vi "Create File Path.vi"(5 "system directory type":T2 caption="시스템 디렉토리 타입" items=["사용자 홈"=0, "사용자 데스크탑"=1, "사용자 문서"=2, "사용자 어플리케이션 데이터"=3, "사용자 환경"=4, "사용자 임시"=5, "퍼블릭 문서"=6, "퍼블릭 어플리케이션 데이터"=7, "퍼블릭 환경"=8, "퍼블릭 캐시"=13, "시스템 코어 라이브러리"=9, "시스템 설치된 라이브러리"=10, "어플리케이션 파일"=11, "부팅 볼륨 루트"=12], 6 "파일타입":T1, 7 "항목":T3=enum."경로생성", 8 "에러 입력":errorcluster caption="에러 입력(에러 없음)", 10 "문자열 in":string, 11 "폴더명 in":path) -> (0 "error out":errorcluster, 1 "파일존재?":bool, 2 "문자열 out":string, 3 "파일경로":path)   [LabVIEW 2020]
uses:
  Controls/Cmd_File path.ctl
  <vilib>/Utility/sysdir.llb/System Directory Type.ctl
  Controls/Cmd_File Type.ctl
  Variables/Global_Cal Info.vi
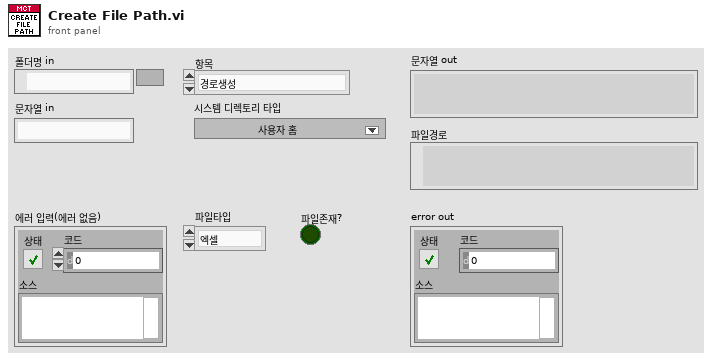
[diagram p1: front panel]
types:
  T1 = typedef "Cmd_File Type.ctl" = enum16{"엑셀", "엑셀(2003)", "텍스트", "설정", "2진", "VI", "CSV", "LOG", "폴더"}
  T2 = typedef "System Directory Type.ctl" = i32
  T3 = typedef "Cmd_File path.ctl" = enum16{"에러로그", "데이터파일경로", "성적서원본", "지난성적서", "Data Files", "경로생성", "Updater", "Template", "설정파일경로", "FTP Upload", "Update 경로", "어플리케이션"}
  T4 = enum32{"invalid app kind", "Development System", "Run Time System", "Student Edition", "Embedded LabVIEW", "Evaluation", "Custom"}
  T5 = cluster{"세부분류코드":string, "형식":string, "옵션":string, "측정기명":string, "EXCEL파일명":string, "TEMP":string}
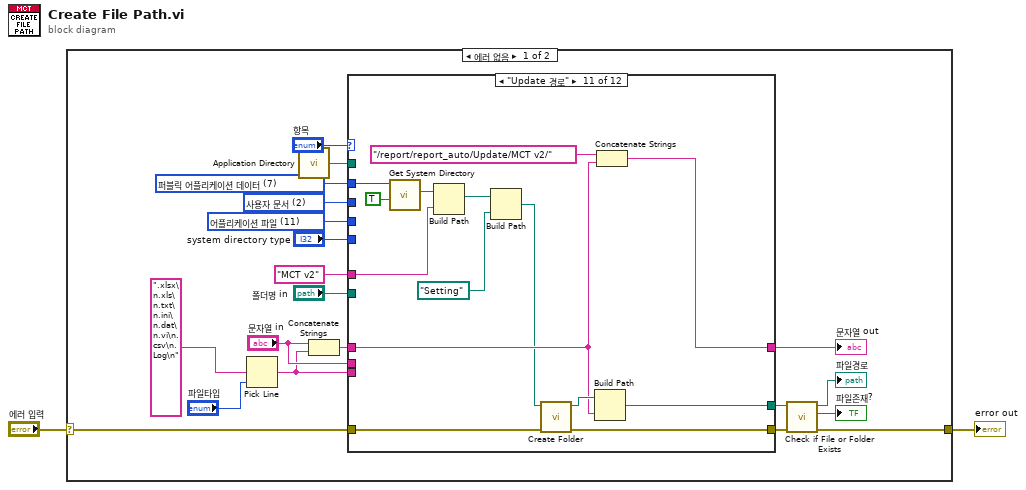
[diagram p0: block diagram]
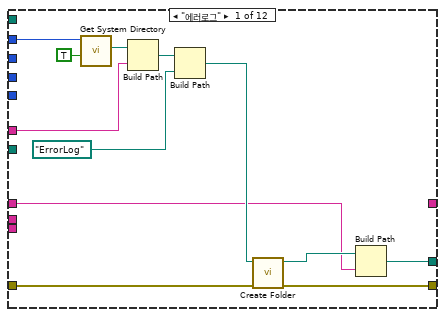
[diagram p2: hidden frame]
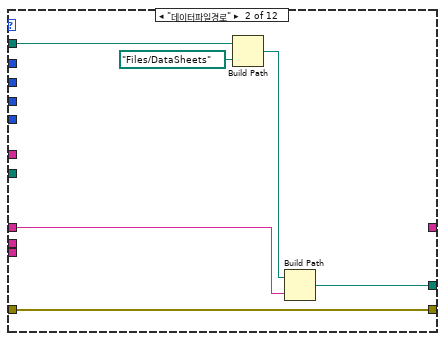
[diagram p3: hidden frame]
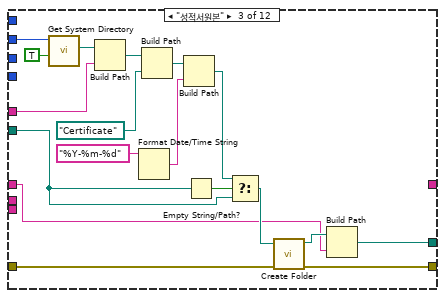
[diagram p4: hidden frame]
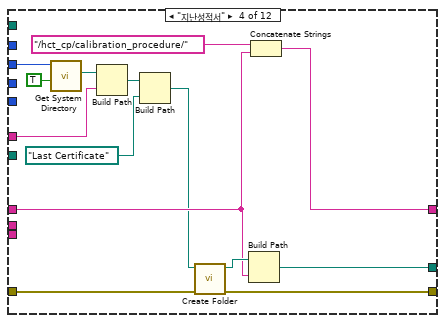
[diagram p5: hidden frame]
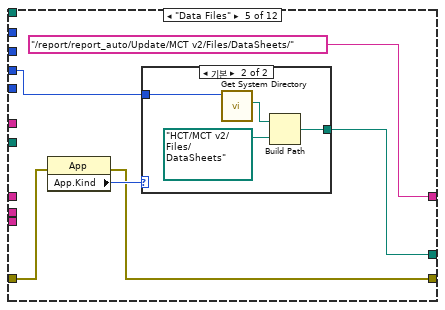
[diagram p6: hidden frame]
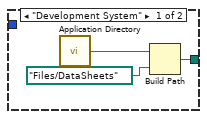
[diagram p7: hidden frame]
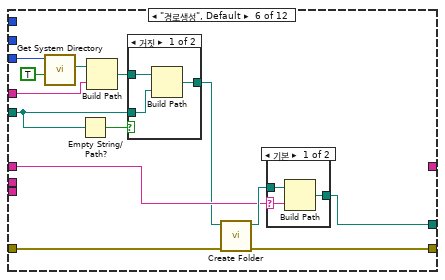
[diagram p8: hidden frame]
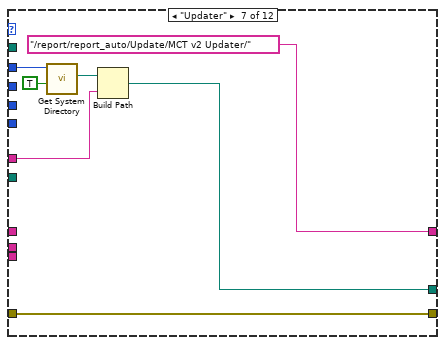
[diagram p11: hidden frame]
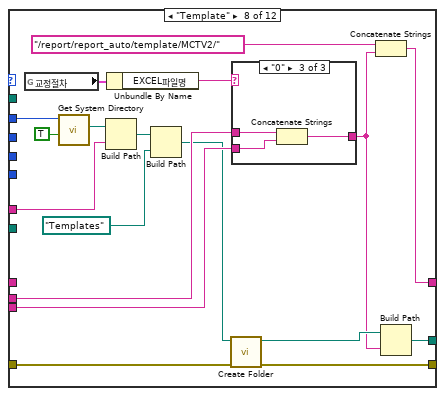
[diagram p12: hidden frame]
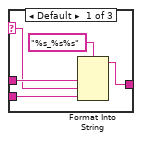
[diagram p13: hidden frame]
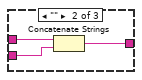
[diagram p14: hidden frame]
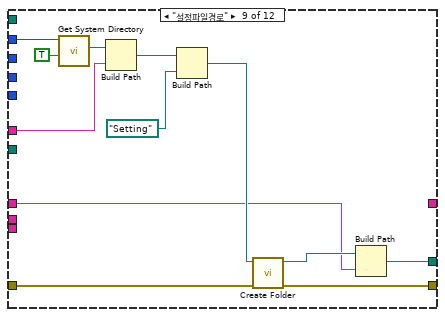
[diagram p15: hidden frame]
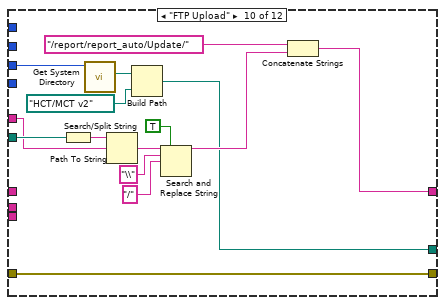
[diagram p16: hidden frame]
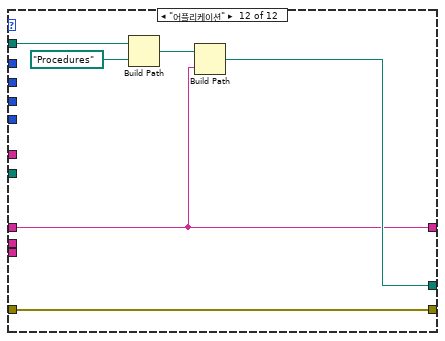
[diagram p17: hidden frame]
diagram:
  n1 = case shown="에러 없음" "에러 입력" {
    selector: "에러 입력" -> [w22 w190]
    tunnel: [w18 w190] -> w1
    frame No Error {
      w4 = T2 11 items=["사용자 홈"=0, "사용자 데스크탑"=1, "사용자 문서"=2, "사용자 어플리케이션 데이터"=3, "사용자 환경"=4, "사용자 임시"=5, "퍼블릭 문서"=6, "퍼블릭 어플리케이션 데이터"=7, "퍼블릭 환경"=8, "퍼블릭 캐시"=13, "시스템 코어 라이브러리"=9, "시스템 설치된 라이브러리"=10, "어플리케이션 파일"=11, "부팅 볼륨 루트"=12] ("system directory type")
      w5 = T2 2 items=["사용자 홈"=0, "사용자 데스크탑"=1, "사용자 문서"=2, "사용자 어플리케이션 데이터"=3, "사용자 환경"=4, "사용자 임시"=5, "퍼블릭 문서"=6, "퍼블릭 어플리케이션 데이터"=7, "퍼블릭 환경"=8, "퍼블릭 캐시"=13, "시스템 코어 라이브러리"=9, "시스템 설치된 라이브러리"=10, "어플리케이션 파일"=11, "부팅 볼륨 루트"=12] ("system directory type 2")
      w7 = T2 7 items=["사용자 홈"=0, "사용자 데스크탑"=1, "사용자 문서"=2, "사용자 어플리케이션 데이터"=3, "사용자 환경"=4, "사용자 임시"=5, "퍼블릭 문서"=6, "퍼블릭 어플리케이션 데이터"=7, "퍼블릭 환경"=8, "퍼블릭 캐시"=13, "시스템 코어 라이브러리"=9, "시스템 설치된 라이브러리"=10, "어플리케이션 파일"=11, "부팅 볼륨 루트"=12] ("system directory type 2")
      n2 = Pick Line(multi-line string=".xlsx\n.xls\n.txt\n.ini\n.dat\n.vi\n.csv\n.Log\n", line index="파일타입") -> (output string=w9:string)  [unwired: 1 in]
      n3 = call <vilib>:"Application Directory.vi"() -> ("Application Directory"=w13:path)
      n4 = Concatenate Strings("문자열 in", w9) -> (w8:string)
      n5 = case shown="\"Update 경로\"" "항목" {
        tunnel: w22 -> [w30 w36 w52 w66 w75 w98 w112 w130 w149 w163 w182 w186]
        tunnel: [w29 w36 w50 w65 w73 w97 w112 w129 w148 w163 w181 w186] -> w20
        tunnel: [w27 w37 w51 w64 w78 w95 w111 w127 w146 w158 w180 w187] -> w21
        tunnel: [_ _ _ w59 "/report/report_auto/Update/MCT v2/Files/DataSheets/" _ "/report/report_auto/Update/MCT v2 Updater/" w115 _ w156 w173 w185] -> w14
        tunnel: "문자열 in" -> [_ _ _ _ _ _ _ w125 _ _ _ _]
        tunnel: w9 -> [_ _ _ _ _ _ _ w124 _ _ _ _]
        tunnel: "폴더명 in" -> [_ _ w43 _ _ w86 _ _ _ w162 _ _]
        tunnel: w13 -> [_ w40 _ _ _ _ _ _ _ _ _ w189]
        tunnel: w8 -> [w25 w35 w48 w63 _ w90 _ _ w144 _ w174 w185]
        tunnel: w7 -> [w23 _ _ _ _ _ w110 w114 w143 _ w176 _]
        tunnel: "MCT v2" ("이름 또는 상대 경로") -> [w32 _ w41 w68 _ w91 w107 w117 w152 w155 w175 _]
        tunnel: w5 -> [_ _ w45 w69 _ _ _ _ _ _ _ _]
        tunnel: w4 -> [_ _ _ _ w77 _ _ _ _ w157 _ _]
        tunnel: "system directory type" -> [_ _ _ _ _ w92 _ _ _ _ _ _]
        frame "에러로그" {
          n6 = call <vilib>:"Get System Directory.vi"("create directory if not found? (F)"=TRUE, "system directory type"=w23) -> ("system directory"=w33:path)  [unwired: 9 in]
          n7 = Build Path(base path=w33, name or relative path=w32) -> (appended path=w31:path)
          n8 = Build Path(base path=w31, name or relative path=path "ErrorLog") -> (appended path=w26:path)
          n9 = call "Create Folder.vi"("에러 입력"=w30, "폴더경로"=w26) -> ("error out"=w29:errorcluster, "dup path"=w28:path)  [unwired: 8 in]
          n10 = Build Path(base path=w28, name or relative path=w25) -> (appended path=w27:path)
        }
        frame "데이터파일경로" {
          n11 = Build Path(base path=w40, name or relative path=path "Files/DataSheets" ("경로")) -> (appended path=w38:path)
          n12 = Build Path(base path=w38, name or relative path=w35) -> (appended path=w37:path)
        }
        frame "성적서원본" {
          n13 = call <vilib>:"Get System Directory.vi"("create directory if not found? (F)"=TRUE, "system directory type"=w45) -> ("system directory"=w46:path)  [unwired: 9 in]
          n14 = Build Path(base path=w46, name or relative path=w41) -> (appended path=w44:path)
          n15 = Format Date/Time String(time format string (%c)="%Y-%m-%d" ("시간 포맷 문자열 (%c)")) -> (date/time string=w58:string)  [unwired: 2 in]
          n16 = Build Path(base path=w44, name or relative path=path "Certificate" ("STD File Path")) -> (appended path=w57:path)
          n17 = Build Path(base path=w57, name or relative path=w58) -> (appended path=w54:path)
          n18 = Empty String/Path?(string/path=w43) -> (empty?=w42:bool)
          n19 = Select(t=w54, s=w42, f=w43) -> (s? t:f=w49:path)
          n20 = call "Create Folder.vi"("에러 입력"=w52, "폴더경로"=w49) -> ("error out"=w50:errorcluster, "dup path"=w53:path)  [unwired: 8 in]
          n21 = Build Path(base path=w53, name or relative path=w48) -> (appended path=w51:path)
        }
        frame "지난성적서" {
          n22 = call <vilib>:"Get System Directory.vi"("create directory if not found? (F)"=TRUE, "system directory type"=w69) -> ("system directory"=w70:path)  [unwired: 9 in]
          n23 = Build Path(base path=w70, name or relative path=w68) -> (appended path=w62:path)
          n24 = Build Path(base path=w62, name or relative path=path "Last Certificate" ("생성할 폴더")) -> (appended path=w60:path)
          n25 = call "Create Folder.vi"("에러 입력"=w66, "폴더경로"=w60) -> ("error out"=w65:errorcluster, "dup path"=w67:path)  [unwired: 8 in]
          n26 = Build Path(base path=w67, name or relative path=w63) -> (appended path=w64:path)
          n27 = Concatenate Strings("/hct_cp/calibration_procedure/", w63) -> (w59:string)
        }
        frame "Data Files" {
          n28 = property class="App"(error in=w75) -> (error out=w73:errorcluster, "App.Kind"=w74:T4)  [unwired: 1 in, 1 out]
          n29 = case shown="기본" w74 {
            tunnel: [w81 w83] -> w78
            tunnel: w77 -> [_ w82]
            frame "Development System" {
              n30 = call <vilib>:"Application Directory.vi"() -> ("Application Directory"=w80:path)
              n31 = Build Path(base path=w80, name or relative path=path "Files/DataSheets" ("이름 또는 상대 경로")) -> (appended path=w81:path)
            }
            frame Default {
              n32 = call <vilib>:"Get System Directory.vi"("system directory type"=w82) -> ("system directory"=w85:path)  [unwired: 10 in]
              n33 = Build Path(base path=w85, name or relative path=path "HCT/MCT v2/Files/DataSheets") -> (appended path=w83:path)
            }
          }
        }
        frame "경로생성", Default {
          n34 = call <vilib>:"Get System Directory.vi"("create directory if not found? (F)"=TRUE, "system directory type"=w92) -> ("system directory"=w93:path)  [unwired: 9 in]
          n35 = Empty String/Path?(string/path=w86) -> (empty?=w87:bool)
          n36 = Build Path(base path=w93, name or relative path=w91) -> (appended path=w89:path)
          n37 = case shown="거짓" w87 {
            tunnel: w89 -> [w101 w102]
            tunnel: [w100 w102] -> w88
            tunnel: w86 -> [w99 _]
            frame False {
              n38 = Build Path(base path=w101, name or relative path=w99) -> (appended path=w100:path)
            }
            frame True {
            }
          }
          n39 = call "Create Folder.vi"("에러 입력"=w98, "폴더경로"=w88) -> ("error out"=w97:errorcluster, "dup path"=w96:path)  [unwired: 8 in]
          n40 = case shown="기본" w90 {
            selector: w90 -> [w103 _]
            tunnel: w96 -> [w105 w106]
            tunnel: [w104 w106] -> w95
            frame Default {
              n41 = Build Path(base path=w105, name or relative path=w103) -> (appended path=w104:path)
            }
            frame "" {
            }
          }
        }
        frame "Updater" {
          n42 = call <vilib>:"Get System Directory.vi"("create directory if not found? (F)"=TRUE, "system directory type"=w110) -> ("system directory"=w113:path)  [unwired: 9 in]
          n43 = Build Path(base path=w113, name or relative path=w107) -> (appended path=w111:path)
        }
        frame "Template" {
          n44 = global read "Global_Cal Info.vi" "교정절차"() -> (w131:T5)
          n45 = call <vilib>:"Get System Directory.vi"("create directory if not found? (F)"=TRUE, "system directory type"=w114) -> ("system directory"=w118:path)  [unwired: 9 in]
          n46 = Build Path(base path=w118, name or relative path=w117) -> (appended path=w116:path)
          n47 = Unbundle By Name(w131) -> ("EXCEL파일명"=w126:string)
          n48 = Build Path(base path=w116, name or relative path=path "Templates" ("생성할 폴더")) -> (appended path=w122:path)
          n49 = call "Create Folder.vi"("에러 입력"=w130, "폴더경로"=w122) -> ("error out"=w129:errorcluster, "dup path"=w128:path)  [unwired: 8 in]
          n50 = case shown="\"0\"" w126 {
            selector: w126 -> [w135 _ _]
            tunnel: w125 -> [w136 w139 w142]
            tunnel: w124 -> [w134 w138 w141]
            tunnel: [w132 w137 w140] -> w120
            frame Default {
              n51 = Format Into String(format string="%s_%s%s" ("포맷 문자열"), w136, w135, w134) -> (resulting string=w132:string)  [unwired: 2 in, 1 out]
            }
            frame "" {
              n52 = Concatenate Strings(w139, w138) -> (w137:string)
            }
            frame "0" {
              n53 = Concatenate Strings(w142, w141) -> (w140:string)
            }
          }
          n54 = Concatenate Strings("/report/report_auto/template/MCTV2/" ("포맷 문자열"), w120) -> (w115:string)
          n55 = Build Path(base path=w128, name or relative path=w120) -> (appended path=w127:path)
        }
        frame "설정파일경로" {
          n56 = call <vilib>:"Get System Directory.vi"("create directory if not found? (F)"=TRUE, "system directory type"=w143) -> ("system directory"=w153:path)  [unwired: 9 in]
          n57 = Build Path(base path=w153, name or relative path=w152) -> (appended path=w151:path)
          n58 = Build Path(base path=w151, name or relative path=path "Setting" ("생성할 폴더")) -> (appended path=w145:path)
          n59 = call "Create Folder.vi"("에러 입력"=w149, "폴더경로"=w145) -> ("error out"=w148:errorcluster, "dup path"=w147:path)  [unwired: 8 in]
          n60 = Build Path(base path=w147, name or relative path=w144) -> (appended path=w146:path)
        }
        frame "FTP Upload" {
          n61 = Path To String(path=w162) -> (string=w164:string)
          n62 = call <vilib>:"Get System Directory.vi"("system directory type"=w157) -> ("system directory"=w159:path)  [unwired: 10 in]
          n63 = Search/Split String(string=w164, search string/char (-)=w155) -> (match + rest of string=w165:string)  [unwired: 1 in, 2 out]
          n64 = Build Path(base path=w159, name or relative path=path "HCT/MCT v2") -> (appended path=w158:path)
          n65 = Search and Replace String(replace all?=TRUE ("모두 대체? (거짓)"), input string=w165, search string="\\" ("검색 문자열"), replace string="/" ("대체 문자열(\"\")")) -> (result string=w169:string)  [unwired: 4 in, 3 out]
          n66 = Concatenate Strings("/report/report_auto/Update/", w169) -> (w156:string)
        }
        frame "Update 경로" {
          n67 = call <vilib>:"Get System Directory.vi"("create directory if not found? (F)"=TRUE, "system directory type"=w176) -> ("system directory"=w177:path)  [unwired: 9 in]
          n68 = Build Path(base path=w177, name or relative path=w175) -> (appended path=w170:path)
          n69 = Build Path(base path=w170, name or relative path=path "Setting" ("생성할 폴더")) -> (appended path=w171:path)
          n70 = call "Create Folder.vi"("에러 입력"=w182, "폴더경로"=w171) -> ("error out"=w181:errorcluster, "dup path"=w183:path)  [unwired: 8 in]
          n71 = Build Path(base path=w183, name or relative path=w174) -> (appended path=w180:path)
          n72 = Concatenate Strings("/report/report_auto/Update/MCT v2/", w174) -> (w173:string)
        }
        frame "어플리케이션" {
          n73 = Build Path(base path=w189, name or relative path=path "Procedures") -> (appended path=w188:path)
          n74 = Build Path(base path=w188, name or relative path=w185) -> (appended path=w187:path)
        }
      }
      "문자열 out" <- w14
      n75 = call <vilib>:"Check if File or Folder Exists.vi"("error in (no error)"=w20, "path"=w21) -> ("error out"=w18:errorcluster, "file or folder exists?"=→"파일존재?":bool, "dup path"=→"파일경로":path)  [unwired: 7 in]
    }
    frame Error {
    }
  }
  "error out" <- w1
